vi "Create Subchannel.vi"() -> (2 "subchannel":T1, 3 "Event Registration Refnum out":refnum<event-registration>)   [LabVIEW 2019, in "Event MessengerM.lvlib" / "EventMessengerMData.lvclass"]
uses:
  EventMessengerMData.lvclass
  EventMessengerMData.lvclass/EventMessengerMData.ctl
  Event Data.ctl
  Event MessengerM.lvlib
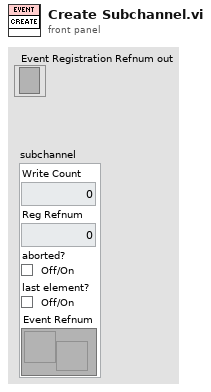
[diagram p1: front panel]
types:
  T1 = cluster{"Write Count":u32, "Reg Refnum":u32, "aborted?":bool, "last element?":bool, "Event Refnum":refnum<user-event>}
  T2 = typedef "Event MessengerM.lvlib/Event Data.ctl" = cluster{"msg":cluster{"cmd":string, "data":variant}, "valid?":bool, "last?":bool, "aborted?":bool}
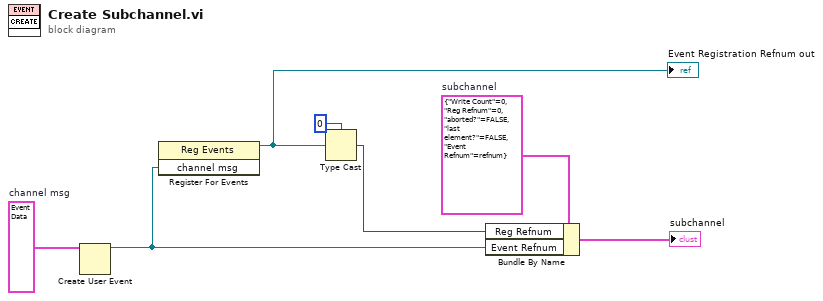
[diagram p0: block diagram]
diagram:
  w2 = T1 {"Write Count"=0, "Reg Refnum"=0, "aborted?"=FALSE, "last element?"=FALSE, "Event Refnum"=refnum}  # subchannel
  w5 = T2 {"msg"={"cmd"="", "data"=variant}, "valid?"=TRUE, "last?"=TRUE, "aborted?"=TRUE}  # channel msg
  n1 = Create User Event(user event datatype=w5) -> (user event=w6:refnum<user-event>)  [unwired: 1 in, 1 out]
  n2 = register-events(w6) -> (reference out=w7:refnum<event-registration>)  [unwired: 2 in, 1 out]
  "Event Registration Refnum out" <- w7
  n3 = Type Cast(type=u32 0 ("Reg Refnum"), x=w7) -> (*(type *) &x=w3:u32)
  n4 = Bundle By Name(cluster=w2, "Reg Refnum"=w3, "Event Refnum"=w6) -> (→"subchannel":T1)
